vi "XP2100_Controller_Manual Test_Main.vi"() -> ()   [LabVIEW 2013]
doc: "This template is for the Queued Message Handler design pattern.\n\nThe Event Handling Loop generates messages based on user interface actions.\n\nThe Message Handling Loop processes messages generated by the Event Handling Loop, or by other messages. The messages are string values, so new messages can be added easily to the Message Cases case structure in the Message Handling Loop. Each message cluster can also provide an optional value for Message Data, which is a variant that can be converted to whatever message-specific data is required."
uses:
  <instrlib>/niHSDIO/niHSDIO.llb/niHSDIO_ctl Voltage Logic Family Values (Ring).ctl
  <instrlib>/niDCPower/nidcpower.llb/niDCPower Sense.ctl
  Controls/Reg_Address_Data.ctl
  Controls/USID.ctl
  controls/UI Data.ctl
  support/Message Queue/Enqueue Message (Single).vi
  support/Message Queue/Enqueue Message (Array).vi
  <vilib>/Utility/error.llb/Error Cluster From Error Code.vi
  <vilib>/ErrorRing/Error Ring.xnode
  support/Message Queue/Message Queue.lvlib
  support/User Event - Stop/User Event - Stop.lvlib
panel:
  in  "Measure":bool=TRUE
  in  "Tab Control":T1(tab)
  in  "HV and PI<0> Settings":T3={"HV SMU Settings"={"Source Range"=0.0001, "Source Limit"=60.0, "Source  limit range"=60.0, "Source level"=0.0, "CH"="0", "Output Enabled"=FALSE, "Source Mode"=enum."Current", "aperture time"=0.001, "sense 2"=1009}, "PI<0>"={"Source Range"=6.0, "Source Limit"=0.01, "Source  limit range"=0.01, "Source level"=1.2, "CH"="0", "Output Enabled"=FALSE, "Source Mode"=enum."Voltage", "aperture time"=0.01666, "sense 2"=1009}} {"PI<0>"."sense 2" items=["Local"=1008, "Remote"=1009]; "PI<0>"."aperture time" format="%#_13p"; "PI<0>"."Source level" format="%#.6p"; "PI<0>"."Source  limit range" format="%#.6p"; "PI<0>"."Source Limit" format="%#.6p"; "PI<0>"."Source Range" format="%#.6p"; "HV SMU Settings"."sense 2" items=["Local"=1008, "Remote"=1009]; "HV SMU Settings"."aperture time" format="%#_13p"; "HV SMU Settings"."Source level" format="%#.6p"; "HV SMU Settings"."Source  limit range" format="%#.6p"; "HV SMU Settings"."Source Limit" format="%#.6p"; "HV SMU Settings"."Source Range" format="%#.6p"}
  in  "DUT and Bridge SMU Settings":T4={"SMU Settings"={"CH"={"voltage level range"=6.0, "current limit"=0.1, "current limit range"=0.1, "voltage level "=1.8, "CH_VIO_BRIDGE"="0", "Output Enabled"=TRUE}, "CH 2"={"voltage level range"=6.0, "current limit"=0.1, "current limit range"=0.1, "voltage level "=1.8, "CH_VSU"="1", "Output Enabled"=TRUE}, "CH 3"={"voltage level range"=6.0, "current limit"=0.1, "current limit range"=0.1, "voltage level "=1.8, "CH_VP"="2", "Output Enabled"=TRUE}, "CH 4"={"voltage level range"=6.0, "current limit"=0.1, "current limit range"=0.1, "voltage level "=1.8, "CH_DUT_VIO"="3", "Output Enabled"=TRUE}}, "sense"=1008, "aperture time"=0.01666} {"aperture time" format="%.2p"; "sense" items=["Local"=1008, "Remote"=1009]; "SMU Settings"."CH 4"."voltage level" format="%#.6p"; "SMU Settings"."CH 4"."current limit range" format="%#.6p"; "SMU Settings"."CH 4"."current limit" format="%#.6p"; "SMU Settings"."CH 4"."voltage level range" format="%#.6p"; "SMU Settings"."CH 3"."voltage level" format="%#.6p"; "SMU Settings"."CH 3"."current limit range" format="%#.6p"; "SMU Settings"."CH 3"."current limit" format="%#.6p"; "SMU Settings"."CH 3"."voltage level range" format="%#.6p"; "SMU Settings"."CH 2"."voltage level" format="%#.6p"; "SMU Settings"."CH 2"."current limit range" format="%#.6p"; "SMU Settings"."CH 2"."current limit" format="%#.6p"; "SMU Settings"."CH 2"."voltage level range" format="%#.6p"; "SMU Settings"."CH"."voltage level" format="%#.6p"; "SMU Settings"."CH"."current limit range" format="%#.6p"; "SMU Settings"."CH"."current limit" format="%#.6p"; "SMU Settings"."CH"."voltage level range" format="%#.6p"}
  in  "Instrument_Visas":T5={"DUT and Bridge Power"="4145_0", "HV_SMU"="4139_1", "PI<0> SMU"="4139_0"}
  in  "HDSIO_Settings":T7={"HSDIO VISA"="6556_0", "Waveform Directory"=path "C:/Users/user/Documents/XP2100/Waveforms", "logic family "=8, "Clock Rate"=20000000.0, "channel list (Clock,Data)"="4,6"} {"Clock Rate" format="%.2p"; "logic family" items=["5.0V Logic"=5, "3.3V Logic"=6, "2.5V Logic"=7, "1.8V Logic"=8, "1.5V Logic"=80, "1.2V Logic"=81]}
  in  "Initialize Instruments":bool
  in  "Update SMU's":bool
  in  "Test Script w_Triggers":bool
  in  "Test Script":string="Script Lowpower\nWait until scriptTrigger0\nGenerate U13LowPower\nend Script"
  in  "RFFE Function":enum16{"Write", "Read"}(ring)
  in  "Reg_Address_Data":T8={"Address"=81, "Data"=0} {"Data" min=1; "Address" format="%.0x"}
  in  "USID":T9 max=15
  out "Read Data":cluster{"USID":u8, "Register":u8, "Data":u8} {"Register" max=31 format="%.0x"; "USID" max=15}
  in  "Run RFFE Waveform":bool
  out "Ext_Read_Reg":i32[](array[numeric])
  out "Ext_Read_Data":u8[](array[numeric])=[31, 144, 7]
  in  "Run Script":bool
  in  "Script Steps":string="Generate\tBRGu8r1Cd64\nWait 200\t\nGenerate\tBRGu8r1Cd57\nWait 200\t\nGenerate\tBRGu8r0d13\nWait 200\t\t\nGenerate\tBRGu8r4d7\nWait 200\t\nGenerate\tBRGu8rCd1\nWait 200\t\nGenerate\tBRGu8r3d32\nWait 200\t\t\nGenerate\tBRGu8r2Bd4\nWait 200\t\nGenerate\tBRGu8r4d103\nWait 200\t\nGenerate\tBRGu8r5d255\nWait 200\t\nGenerate\tBRGu8r6d187\nWait 200\t\nGenerate\tBRGu8r7d6\nWait 200\t\nGenerate\tBRGu8r3d96\nWait 200\t\nGenerate\tBRGu8r4Ad242\nWait 200\t\nGenerate\tBRGu8r4Bd249\nWait 200\t\t\nGenerate\tBRGu8r4Cd254\nWait 200\t\nGenerate\tBRGu8r4Dd244\nWait 200\nGenerate\tBRGu8rC1d253\nWait 200\nGenerate BRGu8rC2d244\nWait 200\n\n"
  out "Dut and Bridge Measurements":T10 {"current measurements" format="%#_6p"}
  out "HV Measurements":T10 {"current measurements" format="%#_6p"}
  out "PI<0> Measurements":T10 {"current measurements" format="%#_6p"}
  in  "Script Notepad: Initialize Bridge":string="Generate\tBRGu8r1Cd64\nWait 20\t\nGenerate\tBRGu8r1Cd57\nWait 20\t\nGenerate\tBRGu8r0d13\nWait 20\t\nGenerate\tBRGu8r4d7\nWait 20\t\nGenerate\tBRGu8rCd1\nWait 20\t\nGenerate\tBRGu8r3d32\nWait 20\t\nGenerate\tBRGu8r2Bd4\nWait 20\t\nGenerate\tBRGu8r4d103\nWait 20\t\nGenerate\tBRGu8r5d255\nWait 20\t\nGenerate\tBRGu8r6d187\nWait 20\t\nGenerate\tBRGu8r7d6\nWait 20\t\nGenerate\tBRGu8r3d96\nWait 20\t\nGenerate\tBRGu8r4Ad242\nWait 20\t\nGenerate\tBRGu8r4Bd249\nWait 20\t\nGenerate\tBRGu8r4Cd254\nWait 20\t\nGenerate\tBRGu8r4Dd244\nWait 20\t\nGenerate\tBRGu8rC1d253\nWait 20\t\nGenerate BRGu8rC2d244\nWait 20\t"
  in  "DUT Info":T11={"Lot #"="", "Wafer #"="", "DUT Coordinates"="", "Comments"="generate HV29"}
  in  "Path":path=path "C:/Users/er080167/Desktop/Delete"
  in  "Save Button":bool
  out "USIDs_Detected":u8[](array[numeric])
  in  "Scan USID's":bool
  out "4_CH_SMU_Settings_Readback":T12(array[cluster]) {"sense 2" items=["Local"=1008, "Remote"=1009]}
  out "HV and PI<0> Instrument Settings Readback":T13={"HV SMU Settings: Readback"={"Source Range"=6.0, "Source Limit"=0.01, "Source  limit range"=0.01, "Source level"=1.2, "CH"="0", "Output Enabled"=FALSE, "Source Mode"=enum."Voltage", "aperture time"=0.01666, "sense 2"=1009}, "PI<0>: Settings Readback"={"Source Range"=6.0, "Source Limit"=0.01, "Source  limit range"=0.01, "Source level"=1.2, "CH"="0", "Output Enabled"=FALSE, "Source Mode"=enum."Voltage", "aperture time"=0.01666, "sense 2"=1009}} {"PI<0>: Settings Readback"."sense 2" items=["Local"=1008, "Remote"=1009]; "PI<0>: Settings Readback"."aperture time" format="%#_13p"; "PI<0>: Settings Readback"."Source level" format="%#.6p"; "PI<0>: Settings Readback"."Source  limit range" format="%#.6p"; "PI<0>: Settings Readback"."Source Limit" format="%#.6p"; "PI<0>: Settings Readback"."Source Range" format="%#.6p"; "HV SMU Settings: Readback"."sense 2" items=["Local"=1008, "Remote"=1009]; "HV SMU Settings: Readback"."aperture time" format="%#_13p"; "HV SMU Settings: Readback"."Source level" format="%#.6p"; "HV SMU Settings: Readback"."Source  limit range" format="%#.6p"; "HV SMU Settings: Readback"."Source Limit" format="%#.6p"; "HV SMU Settings: Readback"."Source Range" format="%#.6p"}
  out "Write or Read":digitalwaveform(graph)={"t0"=timestamp(3585852840.1106524 s since 1904-01-01), "dt"=5e-07, "Y"={"transitions"=[], "data"=[[1, 0, 1, 0], [1, 0, 1, 0], [1, 0, 1, 0], [1, 0, 1, 0], [1, 0, 1, 0], [1, 0, 1, 0], [1, 0, 1, 0], [1, 0, 1, 0], [0, 0, 0, 0], [0, 0, 0, 0], [0, 0, 0, 0], [0, 0, 0, 0], [0, 0, 0, 0], [0, 0, 0, 0], [0, 0, 0, 0], [0, 0, 0, 0], [0, 1, 0, 1], [0, 1, 0, 1], [0, 1, 0, 1], [0, 1, 0, 1], [0, 0, 0, 0], [0, 0, 0, 0], [0, 0, 0, 0], [0, 0, 0, 0], [1, 1, 1, 1], [1, 1, 1, 1], [1, 1, 1, 1], [1, 1, 1, 1], [1, 0, 1, 0], [1, 0, 1, 0], [1, 0, 1, 0], [1, 0, 1, 0], [1, 1, 1, 1], [1, 1, 1, 1], [1, 1, 1, 1], [1, 1, 1, 1], [1, 0, 1, 0], [1, 0, 1, 0], [1, 0, 1, 0], [1, 0, 1, 0], [0, 1, 0, 1], [0, 1, 0, 1], [0, 1, 0, 1], [0, 1, 0, 1], [0, 0, 0, 0], [0, 0, 0, 0], [0, 0, 0, 0], [0, 0, 0, 0], [0, 1, 0, 1], [0, 1, 0, 1], [0, 1, 0, 1], [0, 1, 0, 1], [0, 0, 0, 0], [0, 0, 0, 0], [0, 0, 0, 0], [0, 0, 0, 0], [1, 1, 1, 1], [1, 1, 1, 1], [1, 1, 1, 1], [1, 1, 1, 1], [1, 0, 1, 0], [1, 0, 1, 0], [1, 0, 1, 0], [1, 0, 1, 0], [0, 1, 0, 1], [0, 1, 0, 1], [0, 1, 0, 1], [0, 1, 0, 1], [0, 0, 0, 0], [0, 0, 0, 0], [0, 0, 0, 0], [0, 0, 0, 0], [1, 1, 1, 1], [1, 1, 1, 1], [1, 1, 1, 1], [1, 1, 1, 1], [1, 0, 1, 0], [1, 0, 1, 0], [1, 0, 1, 0], [1, 0, 1, 0], [1, 1, 1, 1], [1, 1, 1, 1], [1, 1, 1, 1], [1, 1, 1, 1], [1, 0, 1, 0], [1, 0, 1, 0], [1, 0, 1, 0], [1, 0, 1, 0], [1, 1, 1, 1], [1, 1, 1, 1], [1, 1, 1, 1], [1, 1, 1, 1], [1, 0, 1, 0], [1, 0, 1, 0], [1, 0, 1, 0], [1, 0, 1, 0], [0, 1, 0, 1], [0, 1, 0, 1], [0, 1, 0, 1], [0, 1, 0, 1], [0, 0, 0, 0], [0, 0, 0, 0], [0, 0, 0, 0], [0, 0, 0, 0], [0, 1, 0, 1], [0, 1, 0, 1], [0, 1, 0, 1], [0, 1, 0, 1], [0, 0, 0, 0], [0, 0, 0, 0], [0, 0, 0, 0], [0, 0, 0, 0], [1, 1, 1, 1], [1, 1, 1, 1], [1, 1, 1, 1], [1, 1, 1, 1], [1, 0, 1, 0], [1, 0, 1, 0], [1, 0, 1, 0], [1, 0, 1, 0], [1, 1, 1, 1], [1, 1, 1, 1], [1, 1, 1, 1], [1, 1, 1, 1], [1, 0, 1, 0], [1, 0, 1, 0], [1, 0, 1, 0], [1, 0, 1, 0], [0, 1, 0, 1], [0, 1, 0, 1], [0, 1, 0, 1], [0, 1, 0, 1], [0, 0, 0, 0], [0, 0, 0, 0], [0, 0, 0, 0], [0, 0, 0, 0], [0, 1, 0, 1], [0, 1, 0, 1], [0, 1, 0, 1], [0, 1, 0, 1], [0, 0, 0, 0], [0, 0, 0, 0], [0, 0, 0, 0], [0, 0, 0, 0], [0, 1, 0, 1], [0, 1, 0, 1], [0, 1, 0, 1], [0, 1, 0, 1], [0, 0, 0, 0], [0, 0, 0, 0], [0, 0, 0, 0], [0, 0, 0, 0], [0, 1, 0, 1], [0, 1, 0, 1], [0, 1, 0, 1], [0, 1, 0, 1], [0, 0, 0, 0], [0, 0, 0, 0], [0, 0, 0, 0], [0, 0, 0, 0], [0, 1, 0, 1], [0, 1, 0, 1], [0, 1, 0, 1], [0, 1, 0, 1], [0, 0, 0, 0], [0, 0, 0, 0], [0, 0, 0, 0], [0, 0, 0, 0], [0, 1, 0, 1], [0, 1, 0, 1], [0, 1, 0, 1], [0, 1, 0, 1], [0, 0, 0, 0], [0, 0, 0, 0], [0, 0, 0, 0], [0, 0, 0, 0], [0, 1, 0, 1], [0, 1, 0, 1], [0, 1, 0, 1], [0, 1, 0, 1], [0, 0, 0, 0], [0, 0, 0, 0], [0, 0, 0, 0], [0, 0, 0, 0], [0, 1, 0, 1], [0, 1, 0, 1], [0, 1, 0, 1], [0, 1, 0, 1], [0, 0, 0, 0], [0, 0, 0, 0], [0, 0, 0, 0], [0, 0, 0, 0], [0, 1, 0, 1], [0, 1, 0, 1], [0, 1, 0, 1], [0, 1, 0, 1], [0, 0, 0, 0], [0, 0, 0, 0], [0, 0, 0, 0], [0, 0, 0, 0], [1, 0, 1, 0], [1, 0, 1, 0], [1, 0, 1, 0], [1, 0, 1, 0], [1, 0, 1, 0], [1, 0, 1, 0], [1, 0, 1, 0], [1, 0, 1, 0], [0, 0, 0, 0], [0, 0, 0, 0], [0, 0, 0, 0], [0, 0, 0, 0], [0, 0, 0, 0], [0, 0, 0, 0], [0, 0, 0, 0], [0, 0, 0, 0], [0, 1, 0, 1], [0, 1, 0, 1], [0, 1, 0, 1], [0, 1, 0, 1], [0, 0, 0, 0], [0, 0, 0, 0], [0, 0, 0, 0], [0, 0, 0, 0], [1, 1, 1, 1], [1, 1, 1, 1], [1, 1, 1, 1], [1, 1, 1, 1], [1, 0, 1, 0], [1, 0, 1, 0], [1, 0, 1, 0], [1, 0, 1, 0], [1, 1, 1, 1], [1, 1, 1, 1], [1, 1, 1, 1], [1, 1, 1, 1], [1, 0, 1, 0], [1, 0, 1, 0], [1, 0, 1, 0], [1, 0, 1, 0], [0, 1, 0, 1], [0, 1, 0, 1], [0, 1, 0, 1], [0, 1, 0, 1], [0, 0, 0, 0], [0, 0, 0, 0], [0, 0, 0, 0], [0, 0, 0, 0], [0, 1, 0, 1], [0, 1, 0, 1], [0, 1, 0, 1], [0, 1, 0, 1], [0, 0, 0, 0], [0, 0, 0, 0], [0, 0, 0, 0], [0, 0, 0, 0], [1, 1, 1, 1], [1, 1, 1, 1], [1, 1, 1, 1], [1, 1, 1, 1], [1, 0, 1, 0], [1, 0, 1, 0], [1, 0, 1, 0], [1, 0, 1, 0], [1, 1, 1, 1], [1, 1, 1, 1], [1, 1, 1, 1], [1, 1, 1, 1], [1, 0, 1, 0], [1, 0, 1, 0], [1, 0, 1, 0], [1, 0, 1, 0], [1, 1, 1, 1], [1, 1, 1, 1], [1, 1, 1, 1], [1, 1, 1, 1], [1, 0, 1, 0], [1, 0, 1, 0], [1, 0, 1, 0], [1, 0, 1, 0], [1, 1, 1, 1], [1, 1, 1, 1], [1, 1, 1, 1], [1, 1, 1, 1], [1, 0, 1, 0], [1, 0, 1, 0], [1, 0, 1, 0], [1, 0, 1, 0], [1, 1, 1, 1], [1, 1, 1, 1], [1, 1, 1, 1], [1, 1, 1, 1], [1, 0, 1, 0], [1, 0, 1, 0], [1, 0, 1, 0], [1, 0, 1, 0], [0, 1, 0, 1], [0, 1, 0, 1], [0, 1, 0, 1], [0, 1, 0, 1], [0, 0, 0, 0], [0, 0, 0, 0], [0, 0, 0, 0], [0, 0, 0, 0], [0, 1, 0, 1], [0, 1, 0, 1], [0, 1, 0, 1], [0, 1, 0, 1], [0, 0, 0, 0], [0, 0, 0, 0], [0, 0, 0, 0], [0, 0, 0, 0], [0, 1, 0, 1], [0, 1, 0, 1], [0, 1, 0, 1], [0, 1, 0, 1], [0, 0, 0, 0], [0, 0, 0, 0], [0, 0, 0, 0], [0, 0, 0, 0], [0, 1, 0, 1], [0, 1, 0, 1], [0, 1, 0, 1], [0, 1, 0, 1], [0, 0, 0, 0], [0, 0, 0, 0], [0, 0, 0, 0], [0, 0, 0, 0], [1, 1, 5, 1], [1, 1, 5, 1], [1, 1, 5, 1], [1, 1, 5, 1], [1, 0, 4, 0], [1, 0, 5, 0], [1, 0, 5, 0], [1, 0, 5, 0], [0, 1, 5, 1], [0, 1, 5, 1], [0, 1, 5, 1], [0, 1, 5, 1], [0, 0, 3, 0], [0, 0, 5, 0], [0, 0, 5, 0], [0, 0, 5, 0], [0, 1, 5, 1], [0, 1, 5, 1], [0, 1, 5, 1], [0, 1, 5, 1], [0, 0, 3, 0], [0, 0, 5, 0], [0, 0, 5, 0], [0, 0, 5, 0], [0, 1, 5, 1], [0, 1, 5, 1], [0, 1, 5, 1], [0, 1, 5, 1], [0, 0, 3, 0], [0, 0, 5, 0], [0, 0, 5, 0], [0, 0, 5, 0], [0, 1, 5, 1], [0, 1, 5, 1], [0, 1, 5, 1], [0, 1, 5, 1], [0, 0, 3, 0], [0, 0, 5, 0], [0, 0, 5, 0], [0, 0, 5, 0], [0, 1, 5, 1], [0, 1, 5, 1], [0, 1, 5, 1], [0, 1, 5, 1], [0, 0, 3, 0], [0, 0, 5, 0], [0, 0, 5, 0], [0, 0, 5, 0], [0, 1, 5, 1], [0, 1, 5, 1], [0, 1, 5, 1], [0, 1, 5, 1], [0, 0, 3, 0], [0, 0, 5, 0], [0, 0, 5, 0], [0, 0, 5, 0], [0, 1, 5, 1], [0, 1, 5, 1], [0, 1, 5, 1], [0, 1, 5, 1], [0, 0, 3, 0], [0, 0, 5, 0], [0, 0, 5, 0], [0, 0, 5, 0], [0, 1, 5, 1], [0, 1, 5, 1], [0, 1, 5, 1], [0, 1, 5, 1], [0, 0, 3, 0], [0, 0, 5, 0], [0, 0, 5, 0], [0, 0, 5, 0], [0, 1, 0, 1], [0, 1, 0, 1], [0, 1, 0, 1], [0, 1, 0, 1], [0, 0, 0, 0], [0, 0, 0, 0], [0, 0, 0, 0], [0, 0, 0, 0]]}}
  out "Display <Replace Me>":string="\"Exit\" button pressed"
  in  "Exit":bool
  # "CH_VIO_BRIDGE"
  # "CH_VSU"
  # "CH_VP"
  # "CH_DUT_VIO"
  # "CH_VIO_BRIDGE"
  # "CH_VSU"
  # "CH_VP"
  # "CH_DUT_VIO"
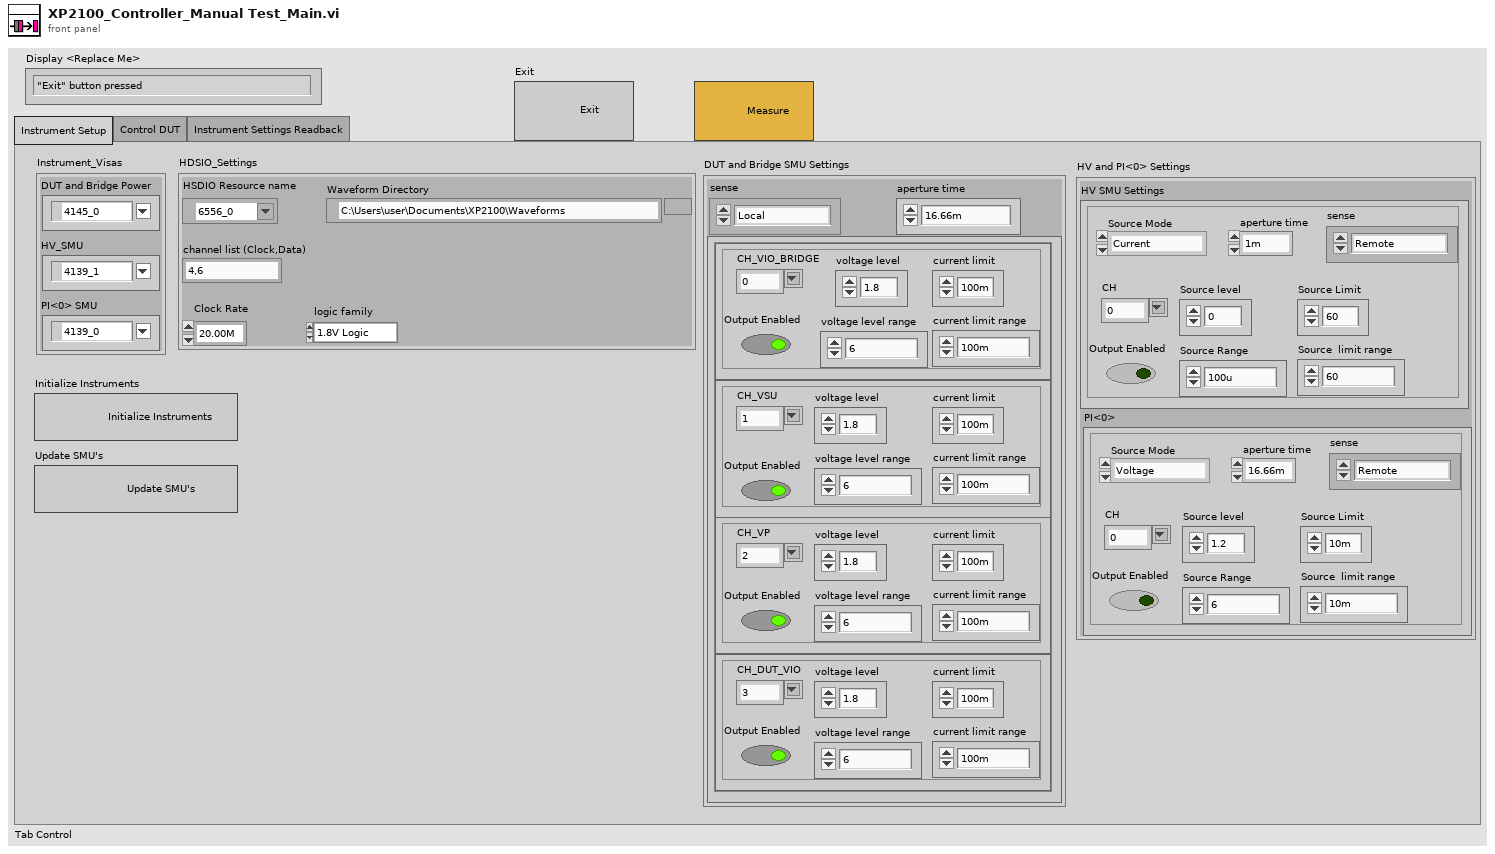
[diagram p1: front panel]
types:
  T1 = enum32{"Instrument Setup", "Control DUT", "Instrument Settings Readback"}
  T2 = typedef "niDCPower Sense.ctl" = i32
  T3 = cluster{"HV SMU Settings":cluster{"Source Range":dbl, "Source Limit":dbl, "Source  limit range":dbl, "Source level":dbl, "CH":string, "Output Enabled":bool, "Source Mode":enum16{"Voltage", "Current"}, "aperture time":dbl, "sense 2":T2}, "PI<0>":cluster{"Source Range":dbl, "Source Limit":dbl, "Source  limit range":dbl, "Source level":dbl, "CH":string, "Output Enabled":bool, "Source Mode":enum16{"Voltage", "Current"}, "aperture time":dbl, "sense 2":T2}}
  T4 = cluster{"SMU Settings":cluster{"CH":cluster{"voltage level range":dbl, "current limit":dbl, "current limit range":dbl, "voltage level ":dbl, "CH_VIO_BRIDGE":string, "Output Enabled":bool}, "CH 2":cluster{"voltage level range":dbl, "current limit":dbl, "current limit range":dbl, "voltage level ":dbl, "CH_VSU":string, "Output Enabled":bool}, "CH 3":cluster{"voltage level range":dbl, "current limit":dbl, "current limit range":dbl, "voltage level ":dbl, "CH_VP":string, "Output Enabled":bool}, "CH 4":cluster{"voltage level range":dbl, "current limit":dbl, "current limit range":dbl, "voltage level ":dbl, "CH_DUT_VIO":string, "Output Enabled":bool}}, "sense":T2, "aperture time":dbl}
  T5 = cluster{"DUT and Bridge Power":refnum<k15>, "HV_SMU":refnum<k15>, "PI<0> SMU":refnum<k15>}
  T6 = typedef "niHSDIO_ctl Voltage Logic Family Values (Ring).ctl" = i32
  T7 = cluster{"HSDIO VISA":refnum<k15>, "Waveform Directory":path, "logic family ":T6, "Clock Rate":dbl, "channel list (Clock,Data)":string}
  T8 = typedef "Reg_Address_Data.ctl" = cluster{"Address":u8, "Data":u8}
  T9 = typedef "USID.ctl" = u8
  T10 = cluster{"voltage measurements":dbl[], "current measurements":dbl[]}
  T11 = cluster{"Lot #":string, "Wafer #":string, "DUT Coordinates":string, "Comments":string}
  T12 = cluster{"Source Range":dbl, "Source Limit":dbl, "Source  limit range":dbl, "Source level":dbl, "CH":string, "Output Enabled":bool, "Source Mode":enum16{"Voltage", "Current"}, "aperture time":dbl, "sense 2":T2}[]
  T13 = cluster{"HV SMU Settings: Readback":cluster{"Source Range":dbl, "Source Limit":dbl, "Source  limit range":dbl, "Source level":dbl, "CH":string, "Output Enabled":bool, "Source Mode":enum16{"Voltage", "Current"}, "aperture time":dbl, "sense 2":T2}, "PI<0>: Settings Readback":cluster{"Source Range":dbl, "Source Limit":dbl, "Source  limit range":dbl, "Source level":dbl, "CH":string, "Output Enabled":bool, "Source Mode":enum16{"Voltage", "Current"}, "aperture time":dbl, "sense 2":T2}}
  T14 = cluster{"HSDIO_ACQ":refnum<k15>, "HSDIO_GEN":refnum<k15>}
  T15 = typedef "UI Data.ctl" = cluster{"Boolean <Replace Me>":bool, "String <Replace Me>":string, "Numeric <Replace Me>":dbl, "Do Something Ref":refnum<vi>, "Do Something Else Ref":refnum<vi>, "Data Display Ref":refnum<vi>, "Exit Button Ref":refnum<vi>}
  T16 = typedef "Message Queue.lvlib/All Message Queues.ctl" = cluster{"UI":refnum<queue>}
  T17 = cluster{"First Reg Address":u8, "Num of Reg to Read":u8}
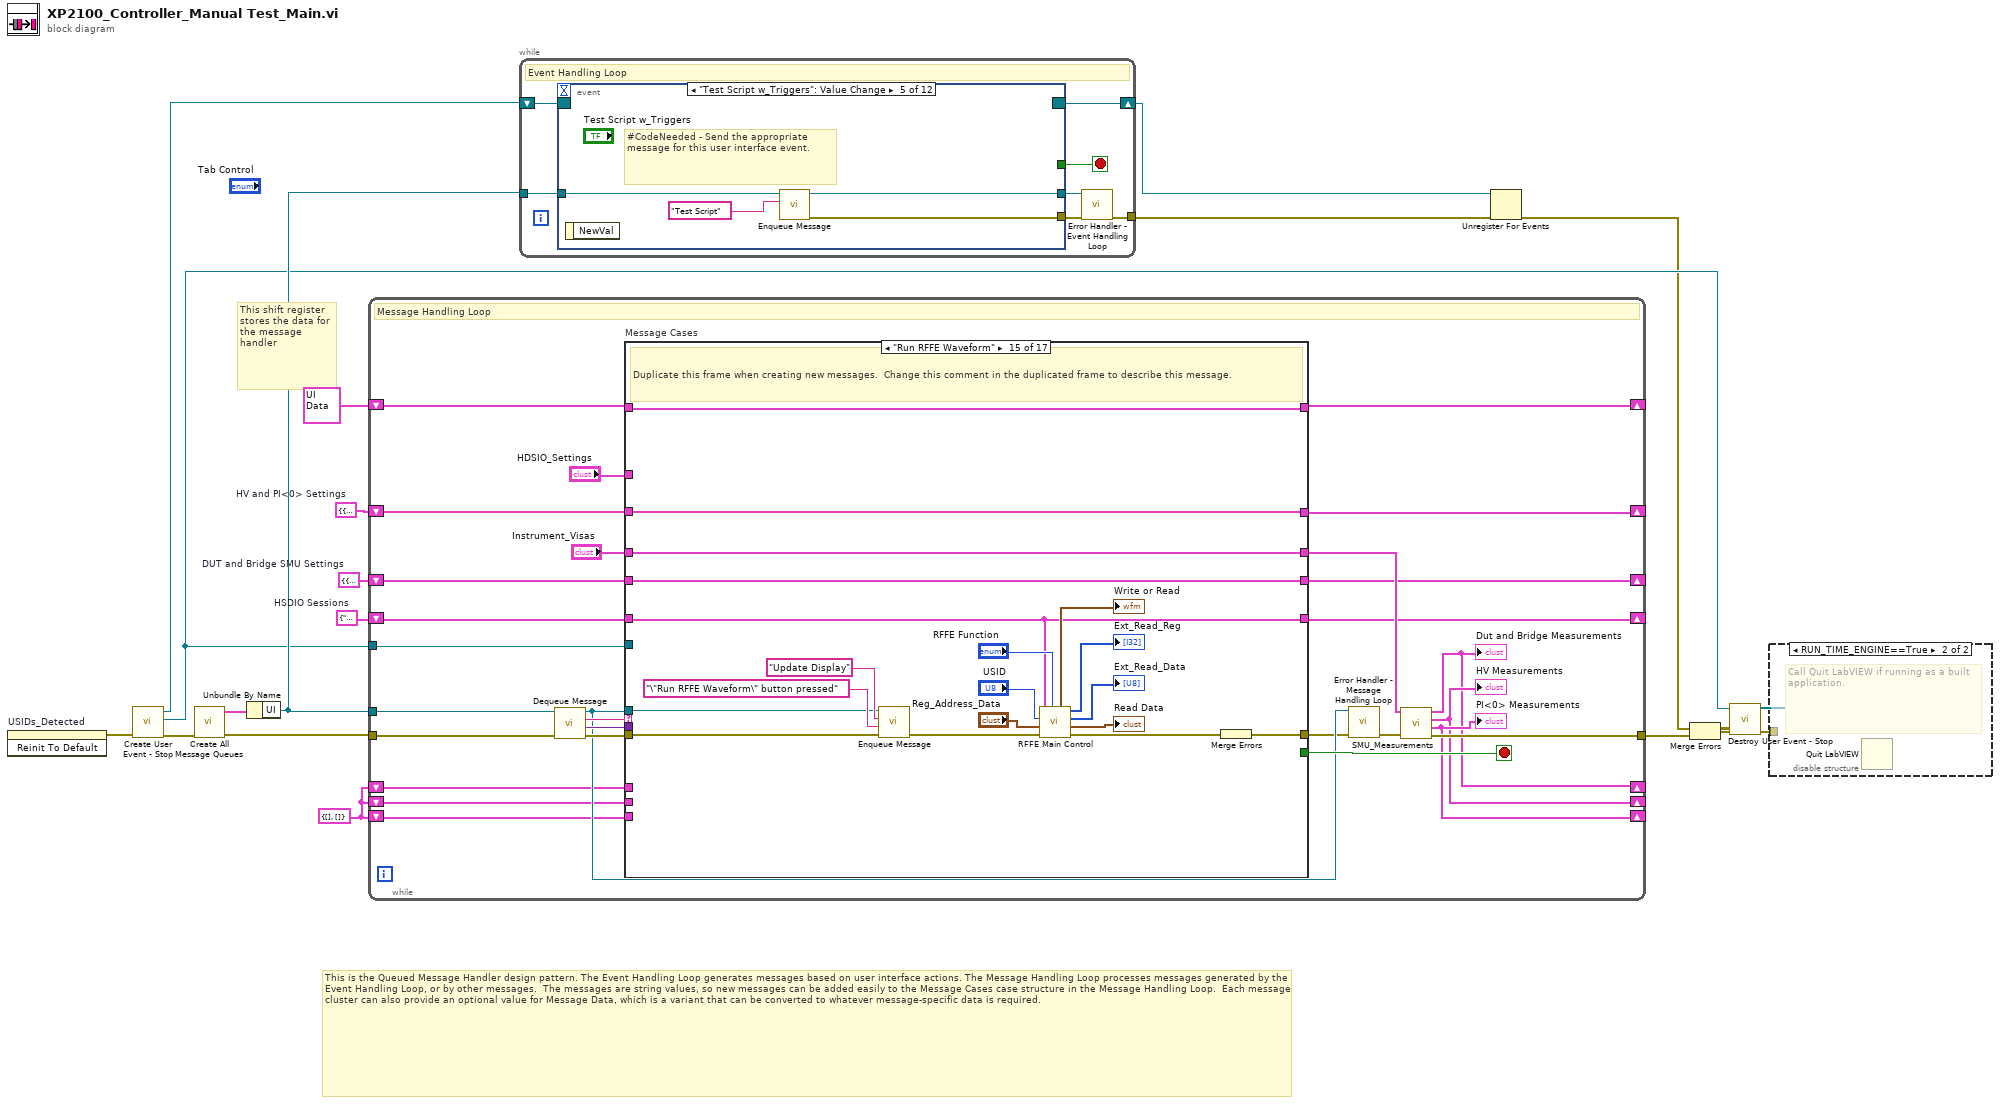
[diagram p0: block diagram]
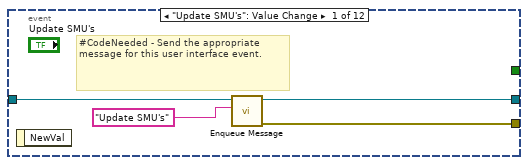
[diagram p3: hidden frame]
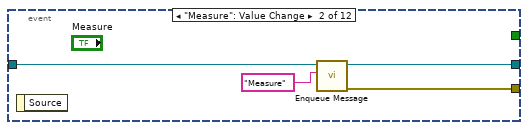
[diagram p4: hidden frame]
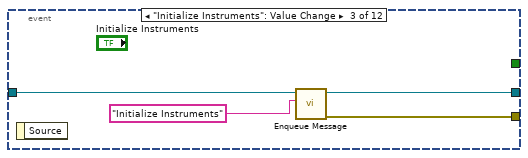
[diagram p5: hidden frame]
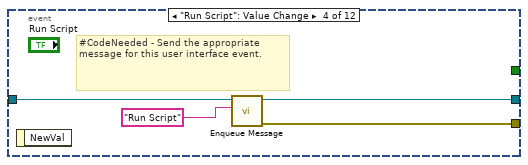
[diagram p6: hidden frame]
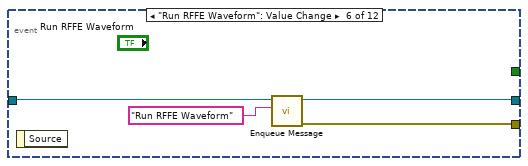
[diagram p7: hidden frame]
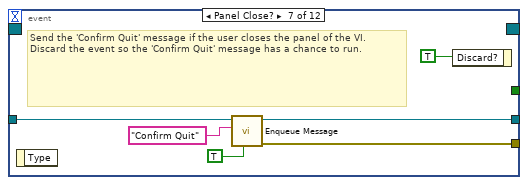
[diagram p8: hidden frame]
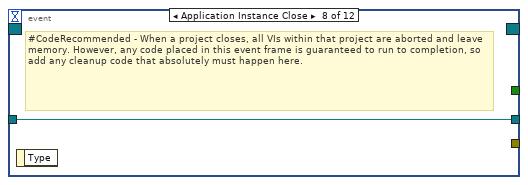
[diagram p9: hidden frame]
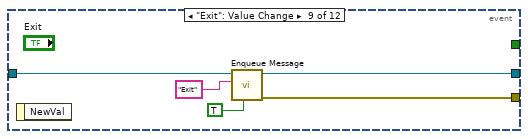
[diagram p10: hidden frame]
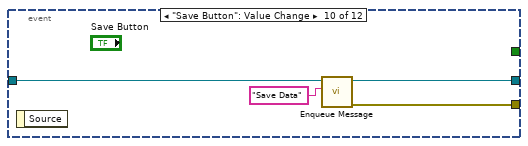
[diagram p11: hidden frame]
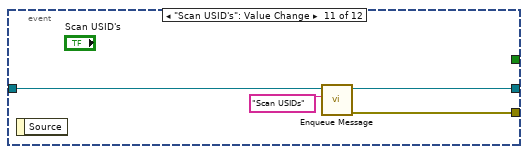
[diagram p12: hidden frame]
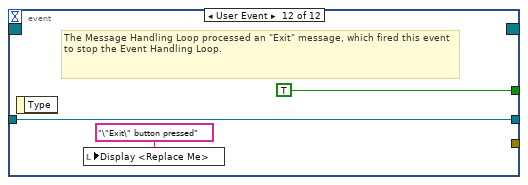
[diagram p13: hidden frame]
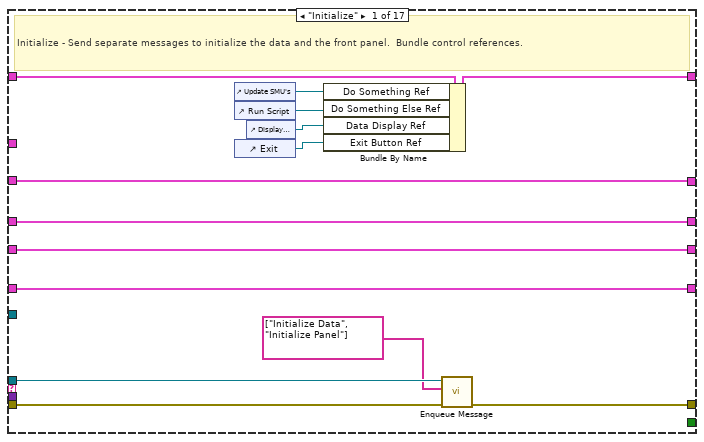
[diagram p14: hidden frame]
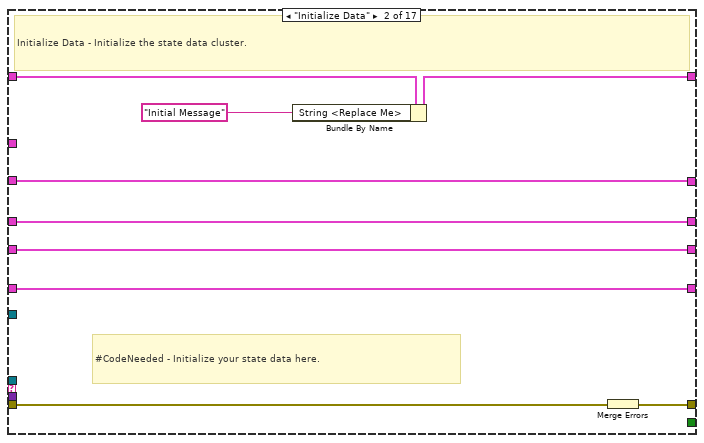
[diagram p15: hidden frame]
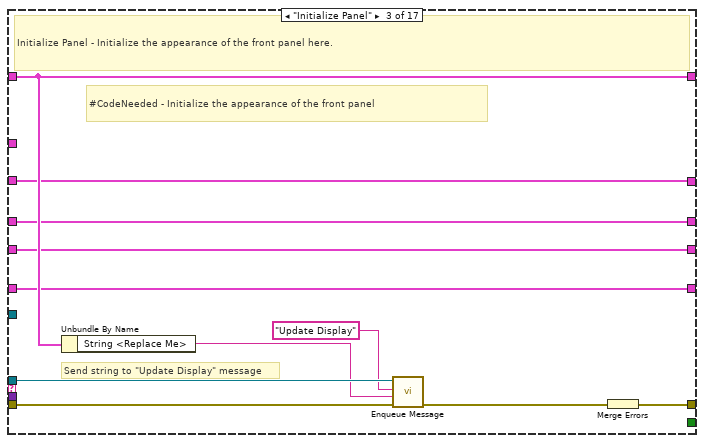
[diagram p16: hidden frame]
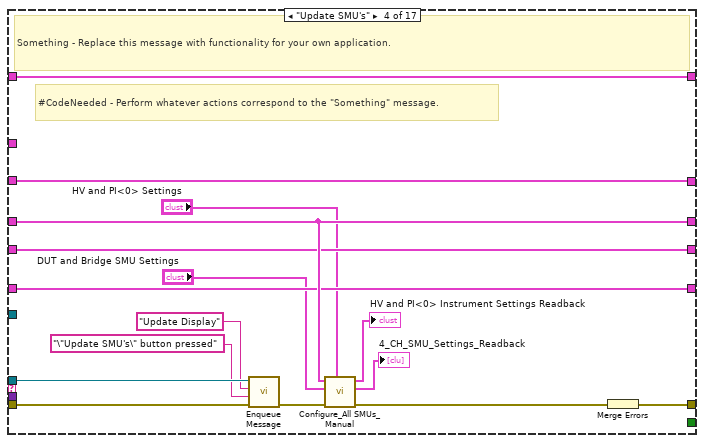
[diagram p17: hidden frame]
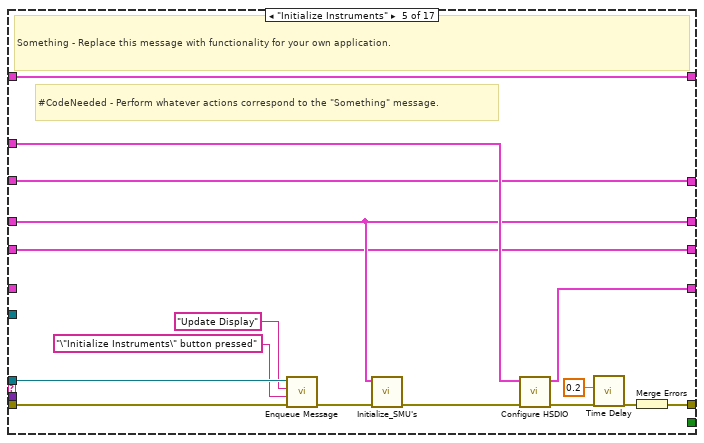
[diagram p18: hidden frame]
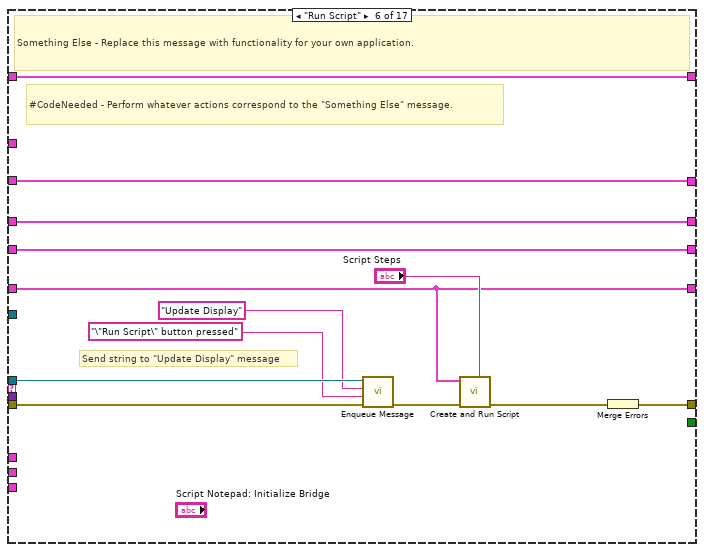
[diagram p19: hidden frame]
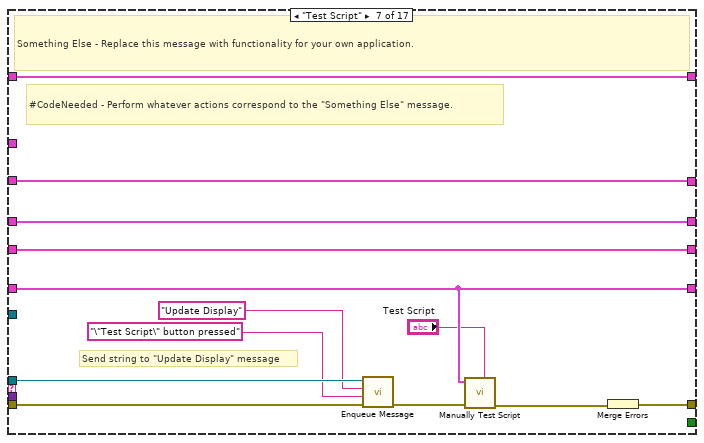
[diagram p20: hidden frame]
diagram:
  w1 = T3 {"HV SMU Settings"={"Source Range"=0.0001, "Source Limit"=60.0, "Source  limit range"=60.0, "Source level"=0.0, "CH"="0", "Output Enabled"=FALSE, "Source Mode"=enum."Current", "aperture time"=0.001, "sense 2"=1009}, "PI<0>"={"Source Range"=6.0, "Source Limit"=0.01, "Source  limit range"=0.01, "Source level"=1.2, "CH"="0", "Output Enabled"=FALSE, "Source Mode"=enum."Voltage", "aperture time"=0.01666, "sense 2"=1009}}  # HV and PI<0> Settings
  w2 = T4 {"SMU Settings"={"CH"={"voltage level range"=0.0, "current limit"=0.0, "current limit range"=0.0, "voltage level "=0.0, "CH_VIO_BRIDGE"="", "Output Enabled"=FALSE}, "CH 2"={"voltage level range"=0.0, "current limit"=0.0, "current limit range"=0.0, "voltage level "=0.0, "CH_VSU"="", "Output Enabled"=FALSE}, "CH 3"={"voltage level range"=0.0, "current limit"=0.0, "current limit range"=0.0, "voltage level "=0.0, "CH_VP"="", "Output Enabled"=FALSE}, "CH 4"={"voltage level range"=0.0, "current limit"=0.0, "current limit range"=0.0, "voltage level "=0.0, "CH_DUT_VIO"="", "Output Enabled"=FALSE}}, "sense"=0, "aperture time"=0.0}  # DUT and Bridge SMU Settings
  w5 = T10 {"voltage measurements"=[], "current measurements"=[]} ("PI<0> Measurements")
  w6 = T14 {"HSDIO_ACQ"="", "HSDIO_GEN"=""}  # HSDIO Sessions
  # "This is the Queued Message Handler design pattern. The Event Handling Loop generates messages based on user interface actions. The Message Handling Loop processes messages generated by the Event Handling Loop, or by other messages.  The messages are string values, so new messages can be added easily to the Message Cases case structure in the Message Handling Loop.  Each message cluster can also provide an optional value for Message Data, which is a variant that can be converted to whatever message-specific data is required."
  # "This shift register stores the data for the message handler"
  n1 = invoke on="USIDs_Detected" class="Arr (strict)" method="Reinit To Default"() -> (error out=w3:errorcluster)  [unwired: 3 in, 2 out]
  n2 = call "Create User Event - Stop.vi"("error in (no error)"=w3) -> ("error out"=w14:errorcluster, "User Event - Stop"=w12:refnum<user-event>, "Stop Event Registration Refnum"=w15:refnum<event-registration>)  [unwired: 8 in]
  n3 = call "Create All Message Queues.vi"("error in (no error)"=w14) -> ("error out"=w4:errorcluster, "Message Queues out"=w18:T16)  [unwired: 9 in]
  n4 = Unbundle By Name(w18) -> ("UI"=w16:refnum<queue>)
  n5 = while {
    tunnel: w16 -> [w38]
    shift-right: [w45] -> _
    shift-left: T15 {"Boolean <Replace Me>"=FALSE, "String <Replace Me>"="", "Numeric <Replace Me>"=0.0, "Do Something Ref"=refnum, "Do Something Else Ref"=refnum, "Data Display Ref"=refnum, "Exit Button Ref"=refnum} ("Data Cluster") -> [w46]
    tunnel: w12 -> [w43]
    tunnel: w4 -> [w42]
    tunnel: [w34] -> w17
    shift-right: [w30] -> _
    shift-left: w6 -> [w29]
    shift-right: [w28] -> _
    shift-left: w5 -> [w23]
    shift-right: [w27] -> _
    shift-left: w5 -> [w24]
    shift-right: [w26] -> _
    shift-left: w5 -> [w25]
    shift-right: [w22] -> _
    shift-left: w2 -> [w21]
    shift-right: [w20] -> _
    shift-left: w1 -> [w19]
    stop <- w44 stop-if-true
    # "Message Handling Loop"
    n6 = call "Dequeue Message.vi"("error in (no error)"=w42, "Message Queue"=w38) -> ("error out"=w41:errorcluster, "Message Data"=w39:variant, "Message"=w40:string, "dup Message Queue"=w37:refnum<queue>)  [unwired: 6 in]
    n7 = case "Message Cases" shown="\"Run RFFE Waveform\"" w40 {
      selector: w40 -> [_ _ _ _ _ _ _ _ _ _ _ _ _ _ _ _ w257]
      tunnel: w37 -> [w58 _ w77 w94 w110 w122 w135 _ w156 w171 _ _ _ _ w233 w252 _]
      tunnel: w41 -> [w59 w69 w78 w91 w107 w123 w136 w147 w164 w175 w182 w189 w203 w215 w234 w248 _]
      tunnel: [w60 w65 w79 w95 w111 w124 w137 w148 w157 w173 w180 w187 w205 w218 w237 w243 w258] -> w36
      tunnel: w46 -> [w57 w68 w80 w96 w112 w125 w138 w149 w163 w174 w181 w188 w206 w219 w238 w251 w259]
      tunnel: [w56 w67 w80 w96 w112 w125 w138 w149 w163 w174 w181 w188 w206 w219 w238 w251 w259] -> w45
      tunnel: [_ _ _ _ _ _ _ _ _ _ _ _ _ _ _ TRUE _] -> w44
      tunnel: w39 -> [_ _ _ _ _ _ _ w146 w162 _ _ _ _ _ _ _ _]
      tunnel: w43 -> [_ _ _ _ _ _ _ _ _ _ _ _ _ _ _ w247 _]
      tunnel: w19 -> [w48 w62 w71 w82 w98 w114 w127 w140 w150 w166 w177 w184 w197 w208 w221 w240 w254]
      tunnel: "Instrument_Visas" -> [w50 w63 w73 w88 w102 w119 w132 w142 w153 w167 w179 w186 w204 w217 w222 w242 w256]
      tunnel: [w50 w63 w73 w88 w102 w119 w132 w142 w153 w167 w179 w186 w204 w217 w222 w242 w256] -> w32
      tunnel: "HDSIO_Settings" -> [_ _ _ _ w106 _ _ _ _ _ _ _ _ _ _ _ _]
      tunnel: [w49 w64 w72 w86 w105 w115 w129 w141 w152 w168 w178 w185 w202 w216 w223 w241 w255] -> w30
      tunnel: w29 -> [w49 w64 w72 w86 _ w115 w129 w141 w152 w168 w178 w185 w202 w216 w223 w241 w255]
      tunnel: w25 -> [_ _ _ _ _ _ _ _ _ _ _ _ _ w211 _ _ _]
      tunnel: w24 -> [_ _ _ _ _ _ _ _ _ _ _ _ _ w210 _ _ _]
      tunnel: w23 -> [_ _ _ _ _ _ _ _ _ _ _ _ _ w209 _ _ _]
      tunnel: [w47 w61 w70 w84 w97 w113 w126 w139 w151 w165 w176 w183 w196 w207 w220 w239 w253] -> w22
      tunnel: w21 -> [w47 w61 w70 w84 w97 w113 w126 w139 w151 w165 w176 w183 w196 w207 w220 w239 w253]
      tunnel: [w48 w62 w71 w82 w98 w114 w127 w140 w150 w166 w177 w184 w197 w208 w221 w240 w254] -> w20
      frame "Initialize" {
        # "Initialize - Send separate messages to initialize the data and the front panel.  Bundle control references."
        n8 = control-ref of="Update SMU's"() -> (w55:refnum<vi>)
        n9 = control-ref of="Run Script"() -> (w54:refnum<vi>)
        n10 = control-ref of="Exit"() -> (w52:refnum<vi>)
        n11 = control-ref of="Display <Replace Me>"() -> (w53:refnum<vi>)
        n12 = Bundle By Name(cluster=w57, "Do Something Ref"=w55, "Do Something Else Ref"=w54, "Data Display Ref"=w53, "Exit Button Ref"=w52) -> (w56:T15)
        n13 = call-poly "Enqueue Message.vi"("error in (no error)"=w59, "Message Array"=string[] ["Initialize Data", "Initialize Panel"], "Message Queue"=w58) -> ("error out"=w60:errorcluster)  [unwired: 7 in, 1 out]
      }
      frame "Initialize Data" {
        # "#CodeNeeded - Initialize your state data here."
        # "Initialize Data - Initialize the state data cluster."
        n14 = Bundle By Name(cluster=w68, "String <Replace Me>"="Initial Message" ("Initial Message")) -> (w67:T15)
        n15 = Merge Errors(w69) -> (w65:errorcluster)
      }
      frame "Initialize Panel" {
        # "Send string to \"Update Display\" message"
        # "#CodeNeeded - Initialize the appearance of the front panel"
        # "Initialize Panel - Initialize the appearance of the front panel here."
        n16 = Unbundle By Name(w80) -> ("String <Replace Me>"=w74:string)
        n17 = call-poly "Enqueue Message.vi"("error in (no error)"=w78, "Message Data"=w74, "Message"="Update Display", "Message Queue"=w77) -> ("error out"=w76:errorcluster)  [unwired: 6 in, 1 out]
        n18 = Merge Errors(w76) -> (w79:errorcluster)
      }
      frame "Update SMU's" {
        # "#CodeNeeded - Perform whatever actions correspond to the \"Something\" message."
        # "Something - Replace this message with functionality for your own application."
        n19 = call-poly "Enqueue Message.vi"("error in (no error)"=w91, "Message Data"="\"Update SMU's\" button pressed" ("\"Do Something\" button pressed"), "Message"="Update Display", "Message Queue"=w94) -> ("error out"=w90:errorcluster)  [unwired: 6 in, 1 out]
        n20 = call "Configure_All SMUs_Manual.vi"("HV and PI<0> Settings"="HV and PI<0> Settings", "Error In"=w90, "DUT and Bridge SMU Settings"="DUT and Bridge SMU Settings", "Instrument_Visas"=w88) -> ("Error Out"=w87:errorcluster, "4_CH_SMu"=→"4_CH_SMU_Settings_Readback":T12, "HV and PI<0> Instrument Settings Readback"=→"HV and PI<0> Instrument Settings Readback":T13)  [unwired: 5 in]
        n21 = Merge Errors(w87) -> (w95:errorcluster)
      }
      frame "Initialize Instruments" {
        # "#CodeNeeded - Perform whatever actions correspond to the \"Something\" message."
        # "Something - Replace this message with functionality for your own application."
        n22 = call-poly "Enqueue Message.vi"("error in (no error)"=w107, "Message Data"="\"Initialize Instruments\" button pressed" ("\"Do Something\" button pressed"), "Message"="Update Display", "Message Queue"=w110) -> ("error out"=w104:errorcluster)  [unwired: 6 in, 1 out]
        n23 = call "Initialize_SMU's.vi"("Error In"=w104, "Instrument_Visas"=w102) -> ("Error Out"=w103:errorcluster)  [unwired: 9 in]
        n24 = call "Configure HSDIO.vi"("error in (no error)"=w103, "HDSIO_Settings"=w106) -> ("error out"=w101:errorcluster, "HSDIO Sessions"=w105:T14)  [unwired: 8 in]
        n25 = call "Time Delay"("error in (no error)"=w101, "Delay Time (s)"=0.2) -> ("error out"=w100:errorcluster)  [unwired: 9 in]
        n26 = Merge Errors(w100) -> (w111:errorcluster)
      }
      frame "Run Script" {
        # "Send string to \"Update Display\" message"
        # "#CodeNeeded - Perform whatever actions correspond to the \"Something Else\" message."
        # "Something Else - Replace this message with functionality for your own application."
        n27 = call-poly "Enqueue Message.vi"("error in (no error)"=w123, "Message Data"="\"Run Script\" button pressed" ("\"Do Something Else\" button pressed"), "Message"="Update Display", "Message Queue"=w122) -> ("error out"=w117:errorcluster)  [unwired: 6 in, 1 out]
        n28 = call "Create and Run Script.vi"("Script Steps"="Script Steps", "Error In"=w117, "HSDIO Sessions"=w115) -> ("Error Out"=w116:errorcluster)  [unwired: 8 in]
        n29 = Merge Errors(w116) -> (w124:errorcluster)
      }
      frame "Test Script" {
        # "Send string to \"Update Display\" message"
        # "#CodeNeeded - Perform whatever actions correspond to the \"Something Else\" message."
        # "Something Else - Replace this message with functionality for your own application."
        n30 = call-poly "Enqueue Message.vi"("error in (no error)"=w136, "Message Data"="\"Test Script\" button pressed" ("\"Do Something Else\" button pressed"), "Message"="Update Display", "Message Queue"=w135) -> ("error out"=w131:errorcluster)  [unwired: 6 in, 1 out]
        n31 = call "Manually Test Script.vi"("Copy Script Into Window"="Test Script", "Error In"=w131, "HSDIO Sessions"=w129) -> ("Error Out"=w130:errorcluster)  [unwired: 8 in]
        n32 = Merge Errors(w130) -> (w137:errorcluster)
      }
      frame "Update Display" {
        # "#CodeRecommended - If you wish to decouple the Message Handling Loop from your user interface, consider creating User Events (like the \"Stop\" event in this VI) to message the Event Handling Loop whenever the user interface needs updating."
        # "Update Display - Convert the message data to a string to display in the Data Display indicator."
        n33 = Variant To Data(error in=w147, type="", Variant=w146) -> (data=→"Display <Replace Me>":string, error out=w144:errorcluster)
        n34 = Merge Errors(w144) -> (w148:errorcluster)
      }
      frame "Error" {
        # "#CodeRecommended - If you ever change the name of this \"Error\" message, you'll need to update the name in the Check Loop Error.vi as well."
        # "#CodeRecommended - This code will always pop up an error dialog and call the 'Exit' message if an error occurs. Add more fine-grained error handling here."
        # "Error - Check the error message data and respond accordingly. This message is sent by the \"Error Handler\" VIs at the end of each loop in this application."
        n35 = Variant To Data(error in=w164, type=errorcluster {"status"=FALSE, "code"=0, "source"=""} ("error constant"), Variant=w162) -> (data=w160:errorcluster, error out=w159:errorcluster)
        n36 = call <vilib>:"Simple Error Handler.vi"("error in (no error)"=w160) -> ()  [unwired: 4 in, 5 out]
        n37 = call-poly "Enqueue Message.vi"("Priority Message? (F)"=TRUE, "Message"="Exit", "Message Queue"=w156) -> ("error out"=w158:errorcluster)  [unwired: 7 in, 1 out]
        n38 = Merge Errors(w158, w159) -> (w157:errorcluster)
      }
      frame "Confirm Quit" {
        # "#CodeNeeded - If you want to provide an \"Are you sure\" dialog (or some other notification) before the application exits, place that code here. This message is typically sent from a Panel Close? event."
        # "Confirm Quit - Message that can confirm whether or not the user wants to exit the application."
        n39 = call-poly "Enqueue Message.vi"("Priority Message? (F)"=TRUE, "error in (no error)"=w175, "Message"="Exit", "Message Queue"=w171) -> ("error out"=w172:errorcluster)  [unwired: 6 in, 1 out]
        n40 = Merge Errors(w172) -> (w173:errorcluster)
      }
      frame "---Copy This Frame---" {
        # "Duplicate this frame when creating new messages.  Change this comment in the duplicated frame to describe this message."
        n41 = Merge Errors(w182) -> (w180:errorcluster)
      }
      frame "Measure" {
        # "Duplicate this frame when creating new messages.  Change this comment in the duplicated frame to describe this message."
        n42 = Merge Errors(w189) -> (w187:errorcluster)
      }
      frame "Scan USIDs" {
        w200 = T9[] [1, 2, 4, 7, 8, 9, 13, 15]  # Potential_USID_Array
        # "USID 8 is Bridge Default"
        # "Duplicate this frame when creating new messages.  Change this comment in the duplicated frame to describe this message."
        n43 = call "Bridge_SCAN_USIDs.vi"("HSDIO Sessions"=w202, "Potential_USID_Array"=w200, "Error In"=w203, "Reg_Address_to_Read"=T17 {"First Reg Address"=31, "Num of Reg to Read"=1}) -> ("USIDs_Detected"=w194:u8[], "Error Out"=w199:errorcluster)  [unwired: 11 in, 3 out]
        "USIDs_Detected" <- w194
        n44 = Search 1D Array(1D array=w194, element=u8 8) -> (index of element=w193:i32)  [unwired: 1 in]
        n45 = Delete From Array(array=w194, index=w193) -> (array with subset deleted=w192:u8[])  [unwired: 1 in, 1 out]
        n46 = Index Array(array=w192, index=0) -> (element=w190:u8)
        n47 = property on="USID" class="DigNum (strict)"(error in=w199, "Value"=w190) -> (error out=w198:errorcluster)  [unwired: 1 in, 1 out]
        n48 = Merge Errors(w198) -> (w205:errorcluster)
      }
      frame "Save Data" {
        # "Duplicate this frame when creating new messages.  Change this comment in the duplicated frame to describe this message."
        n49 = call "Save Data.vi"("PI<0> Measurements"=w209, "HV Measurements"=w210, "Error In"=w215, "Dut and Bridge Measurements"=w211, "DUT Info"="DUT Info", "Path"="Path") -> ("error out"=w214:errorcluster)  [unwired: 5 in]
        n50 = Merge Errors(w214) -> (w218:errorcluster)
      }
      frame "Run RFFE Waveform" {
        # "Duplicate this frame when creating new messages.  Change this comment in the duplicated frame to describe this message."
        n51 = call-poly "Enqueue Message.vi"("error in (no error)"=w234, "Message Data"="\"Run RFFE Waveform\" button pressed" ("\"Do Something Else\" button pressed"), "Message"="Update Display", "Message Queue"=w233) -> ("error out"=w231:errorcluster)  [unwired: 6 in, 1 out]
        n52 = call "RFFE Main Control.vi"("RFFE Function"="RFFE Function", "Error In"=w231, "Reg_Address_Data"="Reg_Address_Data", "USID"="USID", "HSDIO Sessions"=w223) -> ("Error Out"=w232:errorcluster, "Converted Data"=→"Read Data":cluster{"USID":u8, "Register":u8, "Data":u8}, "Data_Readback"=→"Ext_Read_Data":u8[], "Registers_Readback"=→"Ext_Read_Reg":i32[], "HSDIO"=→"Write or Read":digitalwaveform)  [unwired: 2 in]
        n53 = Merge Errors(w232) -> (w237:errorcluster)
      }
      frame "Exit" {
        # "Stop the VI"
        # "Release the message queue reference"
        # "#CodeNeeded - Add any required cleanup code here"
        # "Exit - Exit the application."
        n54 = call "Fire User Event - Stop.vi"("User Event - Stop"=w247) -> ("error out"=w246:errorcluster)  [unwired: 10 in]
        n55 = Release Queue(queue=w252, error in (no error)=w248) -> (error out=w249:errorcluster)  [unwired: 1 in, 2 out]
        n56 = Merge Errors(w246, w249) -> (w245:errorcluster)
        n57 = call "Close_SMU's.vi"("Error In"=w245, "Instrument_Visas"=w242) -> ("Error Out"=w244:errorcluster)  [unwired: 9 in]
        n58 = call "CLOSE_HSDIO.vi"("Error In"=w244, "HSDIO Sessions"=w241) -> ("Error Out"=w243:errorcluster)  [unwired: 9 in]
      }
      frame Default {
        # "'Default' case only runs if there is a message that isn't defined in any of the other cases.  Output a programming error."
        n59 = xnode "Error Ring"("parameter 0"=w257) -> ("error out"=w258:errorcluster)
      }
    }
    n60 = call "Error Handler - Message Handling Loop.vi"("error in (no error)"=w36, "Message Queue"=w37) -> ("dup error in"=w35:errorcluster)  [unwired: 8 in, 1 out]
    n61 = call "SMU_Measurements.vi"("Error In"=w35, "Instrument_Visas"=w32) -> ("Error Out"=w34:errorcluster, "PI<0> Measurements"=w28:T10, "HV Measurements"=w27:T10, "Dut and Bridge Measurements"=w26:T10)  [unwired: 6 in]
    "Dut and Bridge Measurements" <- w26
    "HV Measurements" <- w27
    "PI<0> Measurements" <- w28
  }
  n62 = while {
    tunnel: w16 -> [w273]
    shift-right: [w271] -> w10
    shift-left: w15 -> [w272]
    tunnel: [w267] -> w7
    stop <- w269 stop-if-true
    # "Event Handling Loop"
    n63 = event shown="[4] \"Test Script w_Triggers\": Value Change" {
      selector: w272 -> [_ _ _ _ _ _ _ _ _ _ _ _]
      dyn-events: [_ _ _ _ _ _ _ _ _ _ _ _] -> w271
      timeout: _ -> [_ _ _ _ _ _ _ _ _ _ _ _]
      tunnel: [_ _ _ _ _ _ _ _ _ _ _ TRUE ("Discard?")] -> w269
      tunnel: w273 -> [w277 w281 w284 w289 w293 w296 w302 w304 w309 w313 w317 w320]
      tunnel: [w274 w278 w285 w286 w290 w294 w301 _ w308 w311 w315 _] -> w270
      tunnel: [w276 w280 w283 w288 w292 w295 w300 w304 w307 w312 w316 w320] -> w268
      event "Update SMU's": Value Change {
        # "#CodeNeeded - Send the appropriate message for this user interface event."
        n64 = event-data() -> ()  [unwired: 1 in, 1 out]
        n65 = call-poly "Enqueue Message.vi"("Message"="Update SMU's", "Message Queue"=w277) -> ("error out"=w274:errorcluster, "dup Message Queue"=w276:refnum<queue>)  [unwired: 8 in]
      }
      event "Measure": Value Change {
        n66 = event-data() -> ()  [unwired: 1 in, 1 out]
        n67 = call-poly "Enqueue Message.vi"("Message"="Measure", "Message Queue"=w281) -> ("error out"=w278:errorcluster, "dup Message Queue"=w280:refnum<queue>)  [unwired: 8 in]
      }
      event "Initialize Instruments": Value Change {
        n68 = event-data() -> ()  [unwired: 1 in, 1 out]
        n69 = call-poly "Enqueue Message.vi"("Message"="Initialize Instruments", "Message Queue"=w284) -> ("error out"=w285:errorcluster, "dup Message Queue"=w283:refnum<queue>)  [unwired: 8 in]
      }
      event "Run Script": Value Change {
        # "#CodeNeeded - Send the appropriate message for this user interface event."
        n70 = event-data() -> ()  [unwired: 1 in, 1 out]
        n71 = call-poly "Enqueue Message.vi"("Message"="Run Script", "Message Queue"=w289) -> ("error out"=w286:errorcluster, "dup Message Queue"=w288:refnum<queue>)  [unwired: 8 in]
      }
      event "Test Script w_Triggers": Value Change {
        # "#CodeNeeded - Send the appropriate message for this user interface event."
        n72 = event-data() -> ()  [unwired: 1 in, 1 out]
        n73 = call-poly "Enqueue Message.vi"("Message"="Test Script", "Message Queue"=w293) -> ("error out"=w290:errorcluster, "dup Message Queue"=w292:refnum<queue>)  [unwired: 8 in]
      }
      event "Run RFFE Waveform": Value Change {
        n74 = event-data() -> ()  [unwired: 1 in, 1 out]
        n75 = call-poly "Enqueue Message.vi"("Message"="Run RFFE Waveform", "Message Queue"=w296) -> ("error out"=w294:errorcluster, "dup Message Queue"=w295:refnum<queue>)  [unwired: 8 in]
      }
      event Panel Close? {
        # "Send the 'Confirm Quit' message if the user closes the panel of the VI. Discard the event so the 'Confirm Quit' message has a chance to run."
        n76 = event-data() -> ()  [unwired: 1 in, 1 out]
        n77 = call-poly "Enqueue Message.vi"("Priority Message? (F)"=TRUE, "Message"="Confirm Quit", "Message Queue"=w302) -> ("error out"=w301:errorcluster, "dup Message Queue"=w300:refnum<queue>)  [unwired: 7 in]
        n78 = event-data("Discard?"=TRUE) -> ()  [unwired: 1 in, 1 out]
      }
      event Application Instance Close {
        # "#CodeRecommended - When a project closes, all VIs within that project are aborted and leave memory. However, any code placed in this event frame is guaranteed to run to completion, so add any cleanup code that absolutely must happen here."
        n79 = event-data() -> ()  [unwired: 1 in, 1 out]
      }
      event "Exit": Value Change {
        n80 = event-data() -> ()  [unwired: 1 in, 1 out]
        n81 = call-poly "Enqueue Message.vi"("Priority Message? (F)"=TRUE, "Message"="Exit", "Message Queue"=w309) -> ("error out"=w308:errorcluster, "dup Message Queue"=w307:refnum<queue>)  [unwired: 7 in]
      }
      event "Save Button": Value Change {
        n82 = event-data() -> ()  [unwired: 1 in, 1 out]
        n83 = call-poly "Enqueue Message.vi"("Message"="Save Data", "Message Queue"=w313) -> ("error out"=w311:errorcluster, "dup Message Queue"=w312:refnum<queue>)  [unwired: 8 in]
      }
      event "Scan USID's": Value Change {
        n84 = event-data() -> ()  [unwired: 1 in, 1 out]
        n85 = call-poly "Enqueue Message.vi"("Message"="Scan USIDs", "Message Queue"=w317) -> ("error out"=w315:errorcluster, "dup Message Queue"=w316:refnum<queue>)  [unwired: 8 in]
      }
      event User Event {
        # "The Message Handling Loop processed an \"Exit\" message, which fired this event to stop the Event Handling Loop."
        n86 = event-data() -> ()  [unwired: 1 in, 1 out]
        n87 = local write "Display <Replace Me>"("\"Exit\" button pressed" ("VI Stopped")) -> ()
      }
    }
    n88 = call "Error Handler - Event Handling Loop.vi"("error in (no error)"=w270, "Message Queue"=w268) -> ("dup error in"=w267:errorcluster)  [unwired: 8 in, 1 out]
  }
  n89 = Unregister For Events(event registration refnum=w10, error in=w7) -> (error out=w11:errorcluster)
  n90 = Merge Errors(w11, w17) -> (w13:errorcluster)
  n91 = call "Destroy User Event - Stop.vi"("error in (no error)"=w13, "User Event - Stop"=w12) -> ("error out"=w8:errorcluster)  [unwired: 9 in]
  n92 = disable-structure shown="RUN_TIME_ENGINE==True" {
    disable-tunnel: w8 -> [_ _]
    frame condition #0 (active) {
    }
    frame condition #1 {
      # "Call Quit LabVIEW if running as a built application."
      n93 = Quit LabVIEW() -> ()  [unwired: 1 in]
    }
  }
